vi "Read Swipe.vi"   [LabVIEW 2011, in "LVH-Leap.lvlib"]
uses:
  LVH-Leap.lvlib
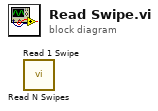
[diagram p0: block diagram]
diagram:
  n1 = call "Read N Swipes.vi"() -> ()  [unwired: 8 in, 4 out]
  n2 = call "Read 1 Swipe.vi"() -> ()  [unwired: 8 in, 4 out]
